vi "Layout Controls.vi"(0 "Controls":refnum<vi>[](array[refnum])) -> (8 "Height":u32)   [LabVIEW 2020, in "TTL XCtrl.xctl"]
uses:
  TTL XCtrl.xctl
panel:
  in  "error in (no error)":errorcluster
  out "error out":errorcluster
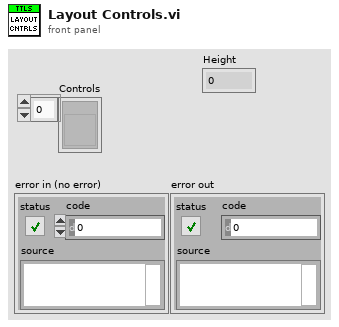
[diagram p1: front panel]
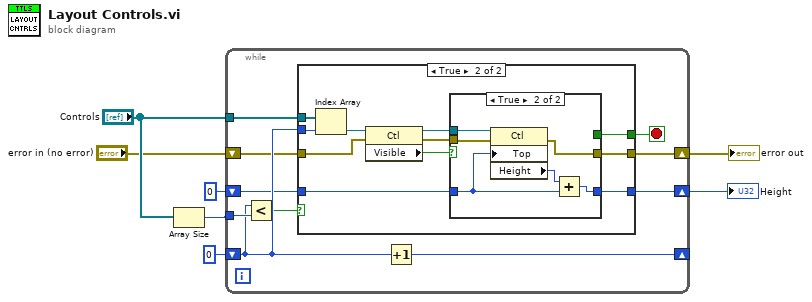
[diagram p0: block diagram]
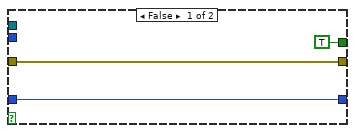
[diagram p2: hidden frame]
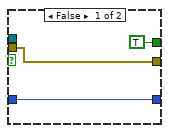
[diagram p3: hidden frame]
diagram:
  n1 = Array Size(array="Controls") -> (size(s)=w7:i32)
  n2 = while {
    shift-right: [w17] -> _
    shift-left: 0 -> [w14]
    tunnel: w7 -> [w16]
    shift-right: [w12] -> w5
    shift-left: 0 -> [w13]
    tunnel: "Controls" -> [w15]
    shift-right: [w8] -> w1
    shift-left: "error in (no error)" -> [w9]
    stop <- w10 stop-if-true
    n3 = Less?(x=w14, y=w16) -> (x < y?=w11:bool)
    n4 = case shown="True" w11 {
      tunnel: w15 -> [_ w31]
      tunnel: w14 -> [_ w30]
      tunnel: w13 -> [w20 w25]
      tunnel: [w20 w24] -> w12
      tunnel: w9 -> [w19 w23]
      tunnel: [w19 w22] -> w8
      tunnel: [TRUE w21] -> w10
      frame False {
      }
      frame True {
        n5 = Index Array(array=w31, index=w30) -> (element=w29:refnum<vi>)
        n6 = property class="Ctl"(reference=w29, error in=w23) -> (reference out=w26:refnum<vi>, error out=w27:errorcluster, "Visible"=w28:bool)
        n7 = case shown="True" w28 {
          tunnel: w27 -> [w33 w39]
          tunnel: w26 -> [_ w40]
          tunnel: w25 -> [w34 w37]
          tunnel: [w34 w36] -> w24
          tunnel: [w33 w35] -> w22
          tunnel: [TRUE _] -> w21
          frame False {
          }
          frame True {
            n8 = property class="Ctl"(reference=w40, error in=w39, "Top"=w37) -> (error out=w35:errorcluster, "Height"=w38:u32)  [unwired: 1 out]
            n9 = Add(x=w38, y=w37) -> (x+y=w36:u32)
          }
        }
      }
    }
    n10 = Increment(x=w14) -> (x+1=w17:i32)
  }
  "error out" <- w1
  "Height" <- w5
